vi "getRampParameters.vi"(8 "error in (no error)":errorcluster, 11 "RampTone in":refnum<class "RampTone.lvclass">) -> (0 "error out":errorcluster, 2 "RampParameters":T1, 3 "RampTone out":refnum<class "RampTone.lvclass">)   [LabVIEW 2009, in "Tools.lvlib" / "Scripting.lvlib" / "RampTone.lvclass"]
uses:
  RampTone.lvclass
  RampTone.lvclass/RampTone.ctl
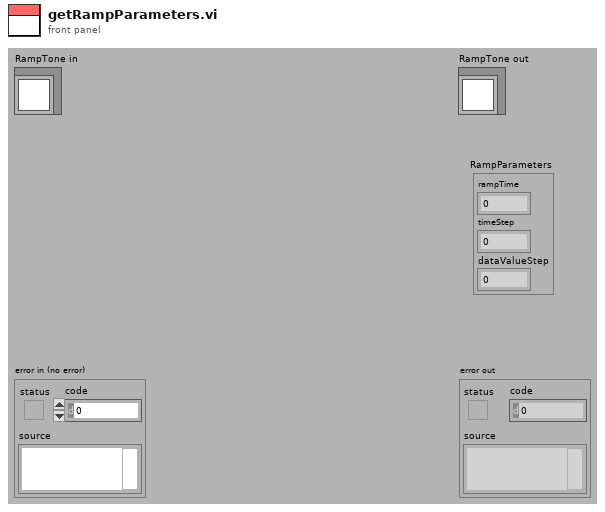
[diagram p1: front panel]
types:
  T1 = cluster{"rampTime":dbl, "timeStep":dbl, "dataValueStep":dbl}
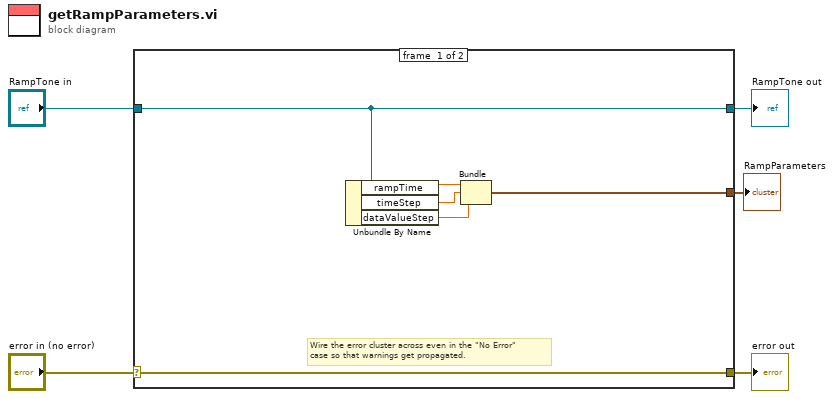
[diagram p0: block diagram]
diagram:
  n1 = case shown="No Error" "error in (no error)" {
    selector: "error in (no error)" -> [w11 w13]
    tunnel: [w11 w13] -> w4
    tunnel: [w10 w12] -> w2
    tunnel: "RampTone in" -> [w10 w12]
    tunnel: [w6 _] -> w1
    frame #0 {
      # "Wire the error cluster across even in the \"No Error\"\ncase so that warnings get propagated."
      n2 = Unbundle By Name(w10) -> ("rampTime"=w9:dbl, "timeStep"=w8:dbl, "dataValueStep"=w7:dbl)
      n3 = Bundle("rampTime"=w9, "timeStep"=w8, "dataValueStep"=w7) -> (w6:T1)  [unwired: 1 in]
    }
    frame #1 {
    }
  }
  "error out" <- w4
  "RampTone out" <- w2
  "RampParameters" <- w1
